vi "Validate and Convert Path.vi"(11 "path":path) -> (3 "validated path as string":string)   [LabVIEW 2019, in "NI_Advanced HTTP Client.lvlib" / "Session.lvclass"]
uses:
  Session.lvclass
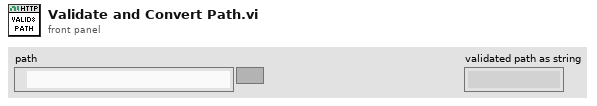
[diagram p1: front panel]
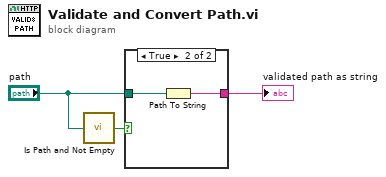
[diagram p0: block diagram]
diagram:
  n1 = call <vilib>:"Is Path and Not Empty.vi"("path"="path") -> ("Is Path and Not Empty?"=w1:bool)  [unwired: 4 in]
  n2 = case shown="True" w1 {
    tunnel: [_ w5] -> w3
    tunnel: "path" -> [_ w4]
    frame False {
    }
    frame True {
      n3 = Path To String(path=w4) -> (string=w5:string)
    }
  }
  "validated path as string" <- w3
